vi "vipm_InstallVIP.vi"(8 "error in (no error)":errorcluster, 11 "CommandLine":string[](array[string])) -> (0 "error out":errorcluster, 2 "test details":string, 3 "output to action":string)   [LabVIEW 2014]
uses:
  <userlib>/_OpenG.lib/file/file.llb/File Exists - Scalar__ogtk.vi
  <userlib>/_OpenG.lib/string/string.llb/Trim Whitespace (String)__ogtk.vi
  <vilib>/JKI/VIPM API/VIPM API_vipm_api.lvlib
  _lvcicd/_lvcicd_support_2014.lvlib
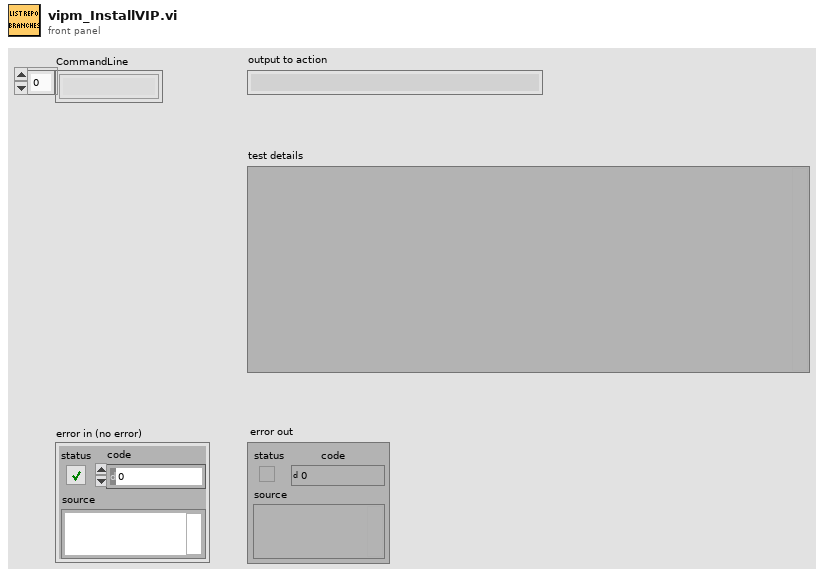
[diagram p1: front panel]
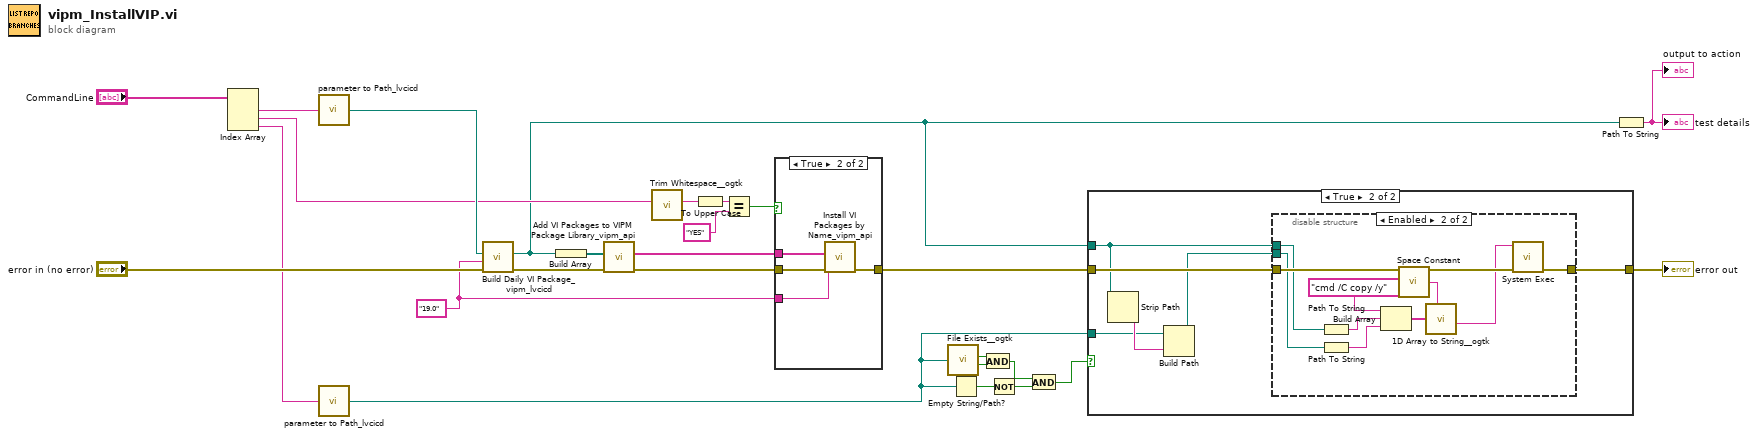
[diagram p0: block diagram]
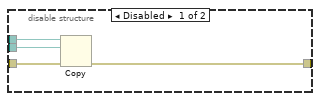
[diagram p3: hidden frame]
diagram:
  w20 = "19.0" ("LabVIEW Version")
  n1 = Index Array(array="CommandLine") -> (element #1=w24:string, element #2=w15:string, element #3=w10:string)  [unwired: 3 in]
  n2 = call "parameter to Path_lvcicd.vi"("String"=w24) -> ("Path"=w26:path)
  n3 = call "parameter to Path_lvcicd.vi"("String"=w10) -> ("Path"=w11:path)
  n4 = call "Build Daily VI Package_vipm_lvcicd.vi"("error in (no error)"="error in (no error)", "LabVIEW Version"=w20, "vipb"=w26) -> ("error out"=w21:errorcluster, "Build Output"=w8:path)  [unwired: 5 in, 2 out]
  n5 = Build Array(w8) -> (w22:path[])
  n6 = call <vilib>:"Add VI Packages to VIPM Package Library_vipm_api.vi"("error in (no error)"=w21, "Packages to add to VIPM Library (vipc,vip,ogp)"=w22) -> ("error out"=w19:errorcluster, "Package Names Added"=w18:string[])  [unwired: 8 in]
  n7 = call-poly <userlib>:"Trim Whitespace__ogtk.vi"("String in"=w15) -> ("String out"=w12:string)  [unwired: 6 in]
  n8 = To Upper Case(1:w12) -> (0:w13:string)
  n9 = Equal?(x=w13, y="YES") -> (x = y?=w16:bool)
  n10 = case shown="True" w16 {
    tunnel: w19 -> [w27 w31]
    tunnel: [w27 w30] -> w17
    tunnel: w20 -> [_ w29]
    tunnel: w18 -> [_ w28]
    frame False {
    }
    frame True {
      n11 = call <vilib>:"Install VI Packages by Name_vipm_api.vi"("error in (no error)"=w31, "LabVIEW Version"=w29, "Package Names to Install []"=w28) -> ("error out"=w30:errorcluster)  [unwired: 8 in]
    }
  }
  n12 = call-poly <userlib>:"File Exists__ogtk.vi"("file path"=w11) -> ("is directory"=w7:bool, "exists"=w6:bool)  [unwired: 6 in]
  n13 = Empty String/Path?(string/path=w11) -> (empty?=w5:bool)
  n14 = And(x=w7, y=w6) -> (x .and. y?=w4:bool)
  n15 = Not(x=w5) -> (.not. x?=w2:bool)
  n16 = And(x=w4, y=w2) -> (x .and. y?=w3:bool)
  n17 = case shown="True" w3 {
    tunnel: w17 -> [w32 w38]
    tunnel: [w32 w37] -> w9
    tunnel: w8 -> [_ w35]
    tunnel: w11 -> [_ w33]
    frame False {
    }
    frame True {
      n18 = Strip Path(path=w35) -> (name=w34:string)  [unwired: 1 out]
      n19 = Build Path(base path=w33, name or relative path=w34) -> (appended path=w36:path)
      n20 = disable-structure shown="Enabled" {
        disable-tunnel: w38 -> [w42 w51]
        disable-tunnel: [w41 w52] -> w37
        disable-tunnel: w36 -> [w40 w49]
        disable-tunnel: w35 -> [w39 w50]
        frame Disabled {
          n21 = Copy(8:w42, 10:w40, 11:w39) -> (0:w41:errorcluster)  [unwired: 2 in, 2 out]
        }
        frame Enabled {
          n22 = Path To String(path=w50) -> (string=w47:string)
          n23 = Path To String(path=w49) -> (string=w46:string)
          n24 = Build Array("cmd /C copy /y" ("name"), w47, w46) -> (w45:string[])
          n25 = call <vilib>:"Space Constant.vi"() -> ("String"=w44:string)
          n26 = call <userlib>:"1D Array to String__ogtk.vi"("delimiter (Tab)"=w44, "Array of Strings"=w45) -> ("delimited string"=w43:string)  [unwired: 9 in]
          n27 = call <vilib>:"System Exec.vi"("error in (no error)"=w51, "command line"=w43) -> ("error out"=w52:errorcluster)  [unwired: 6 in, 3 out]
        }
      }
    }
  }
  "error out" <- w9
  n28 = Path To String(path=w8) -> (string=→"test details" →"output to action":string)
